vi "000_LaunchPanel.vi"(11 "Queue Ref In":T1={"UI"=refnum, "Message"=refnum, "Data"=refnum, "Caller"=refnum, "Name"="000 Common", "Data Path"=path "", "Class Path"=path "", "SubPanel"=refnum, "Project Name"="", "MNT"="", "Title"="", "Data Source"=refnum, "Queue List"={}, "VI"=refnum, "UE"=refnum}) -> ()   [LabVIEW 2020]
doc: "000001"
uses:
  Alin/QMH/000 Module Data Type.ctl
  Alin/QMH/Queue Message.ctl
panel:
  out "Tips":string
  out "Title":u8(slide) scale=0.0..100.0
  # "欢迎使用AlinFramework"
  # "加油小林哥Bilibili"
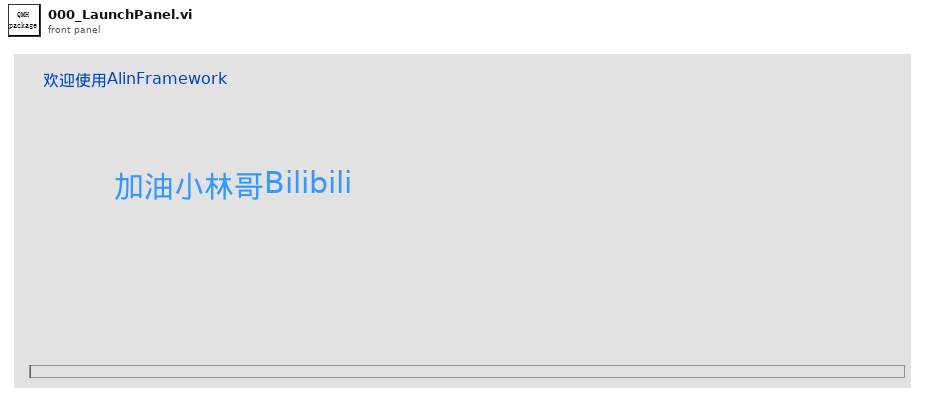
[diagram p1: front panel]
types:
  T1 = typedef "000 Module Data Type.ctl" = cluster{"UI":refnum<queue>, "Message":refnum<queue>, "Data":refnum<queue>, "Caller":refnum<queue>, "Name":string, "Data Path":path, "Class Path":path, "SubPanel":refnum<vi>, "Project Name":string, "MNT":string, "Title":string, "Data Source":refnum<queue>, "Queue List":map{string, refnum<queue>}, "VI":refnum<vi>, "UE":refnum<user-event>}
  T2 = cluster{"Queue":T1, "Delay":cluster{"Count Time(ms)":u32, "Delay Time(ms)":u32, "Next":string, "Restart":bool}}
  T3 = enum32{"Invalid", "Standard", "Closed", "Hidden", "Minimized", "Maximized"}
  T4 = typedef "eventvkey.ctl" = enum16{"ASCII", "Enter", "Return", "Shift", "Ctrl", "Alt", "Cmd", "Opt", "Caps", "NumLock", "Clear", "Break", "Up", "Down", "Left", "Right", "Insert", "Delete", "Home", "End", "PageUp", "PageDown", "Escape", "Help", "Pause", "ScrollLock", "F1", "F2", "F3", "F4", "F5", "F6", "F7", "F8", "F9", "F10", "F11", "F12", "F13", "F14", "F15", "F16", "F17", "F18", "F19", "F20", "F21", "F22", "F23", "F24", "Play", "VolumeUp", "VolumeDown", "Mute", "Two Byte Char"}
  T5 = cluster{"Shift":bool, "Ctrl":bool, "Alt":bool, "Cmd":bool, "Opt":bool}
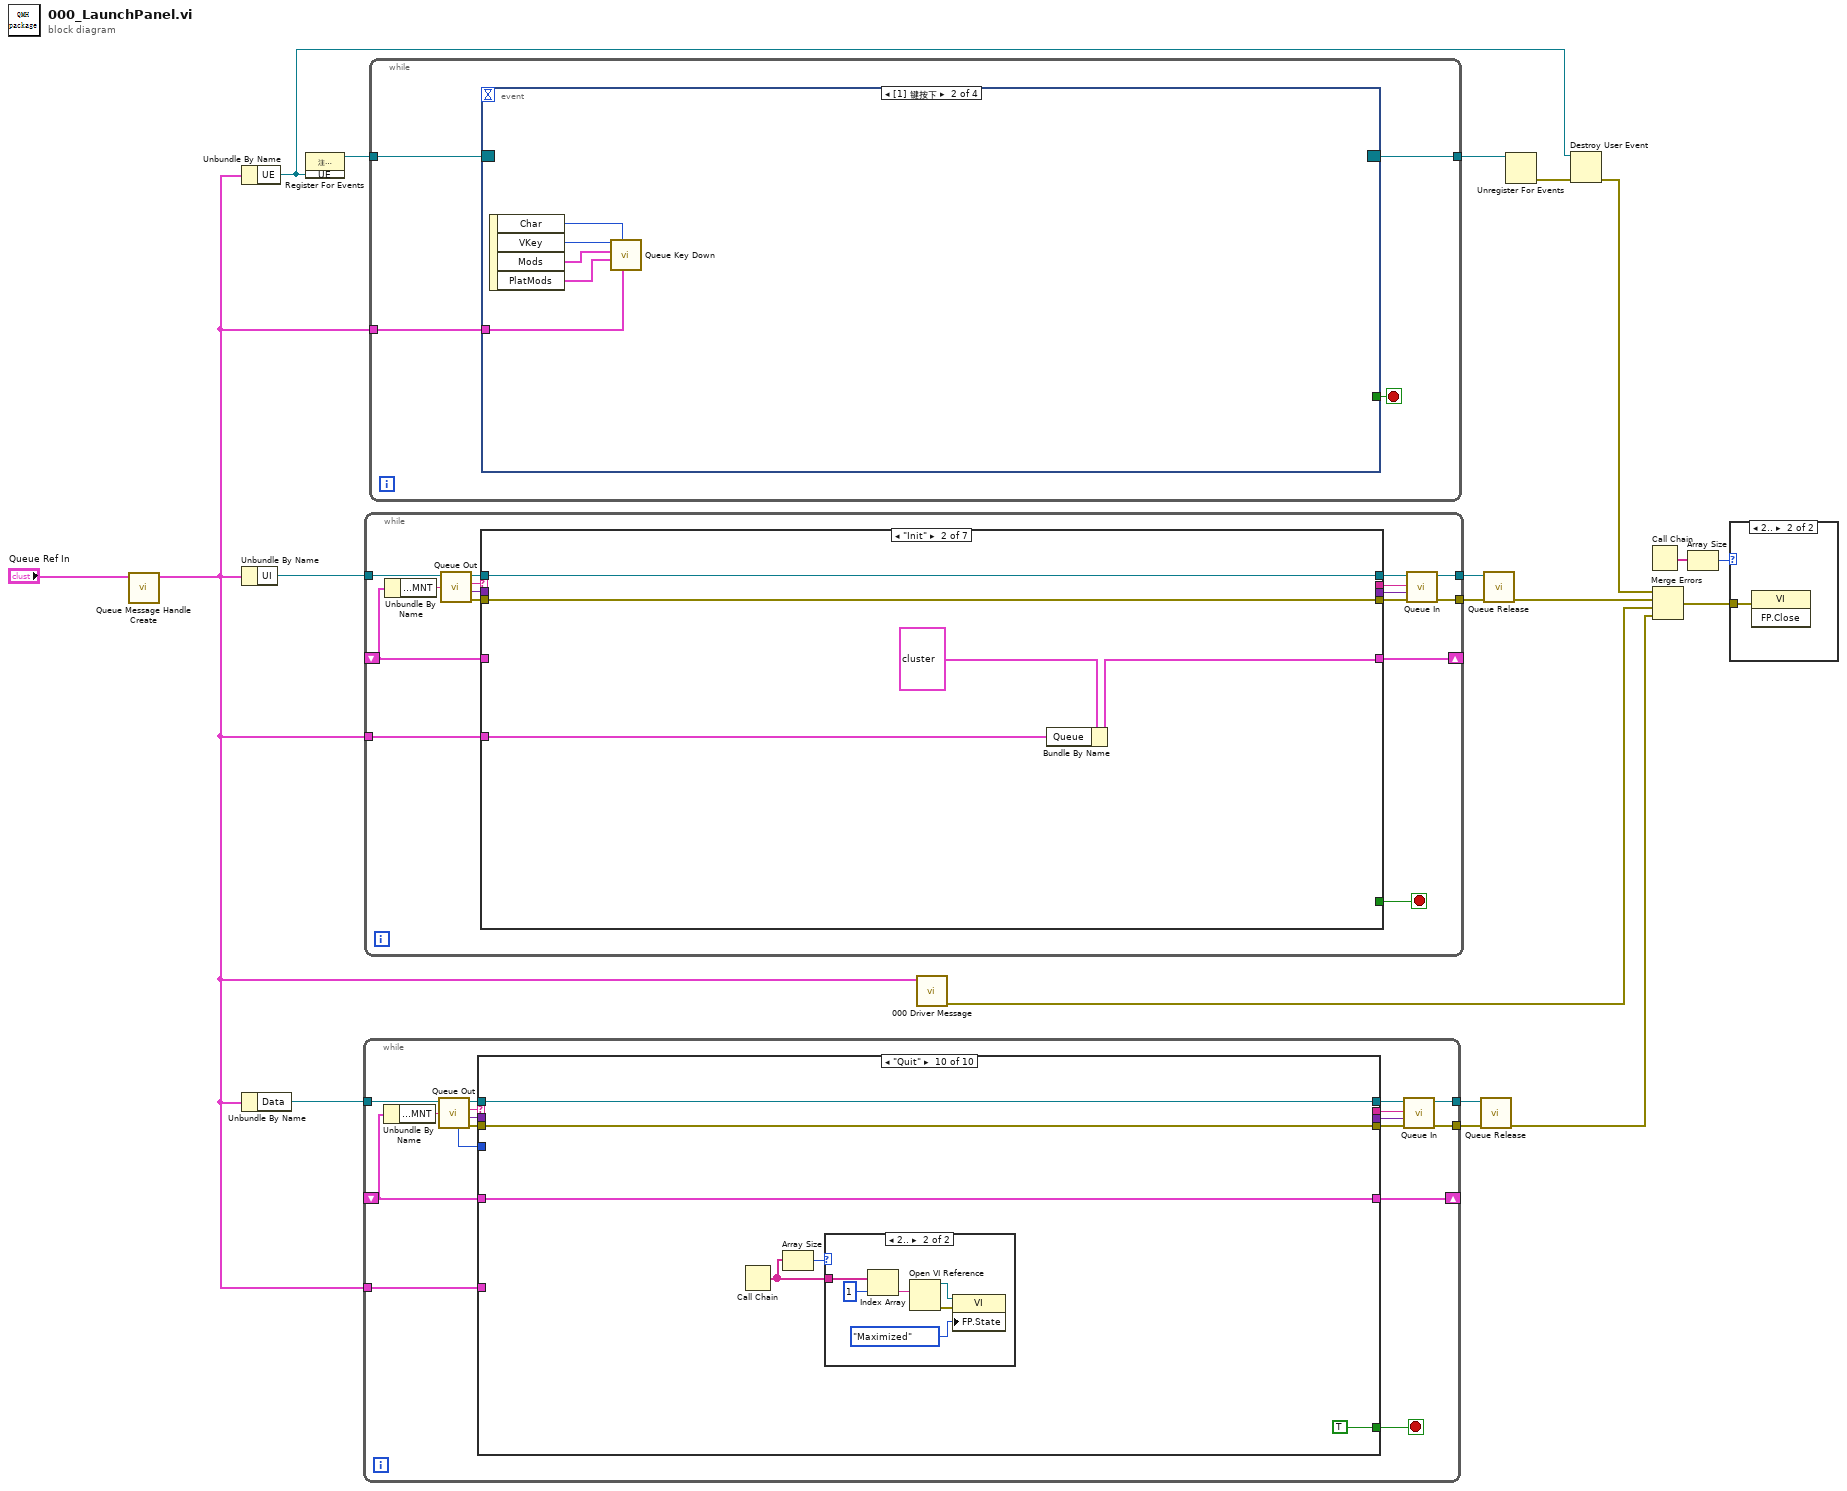
[diagram p0: block diagram]
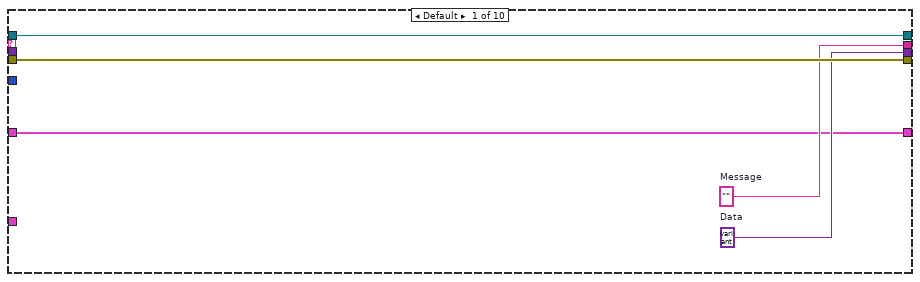
[diagram p2: hidden frame]
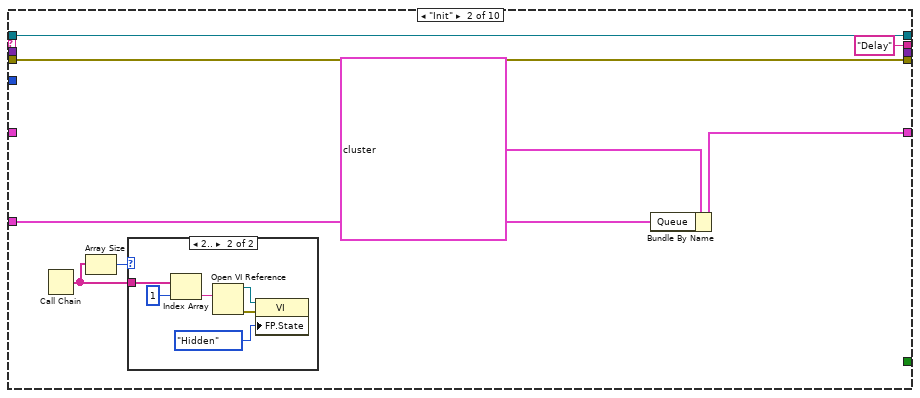
[diagram p3: hidden frame]
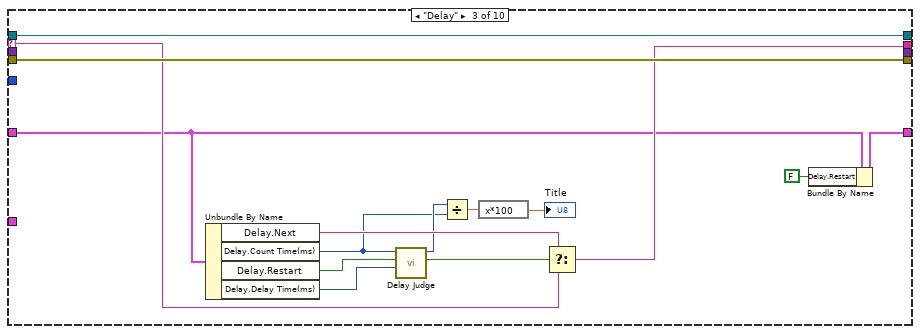
[diagram p5: hidden frame]
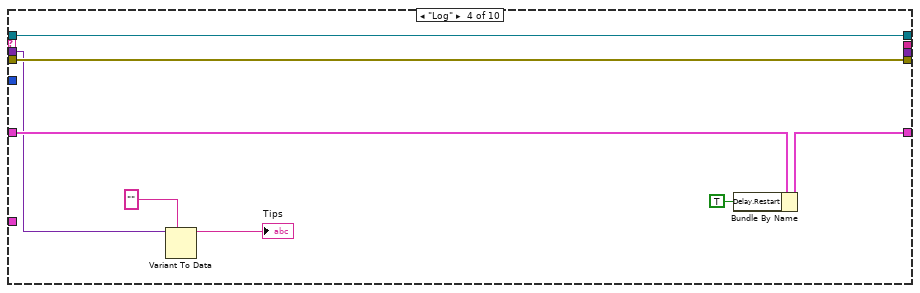
[diagram p6: hidden frame]
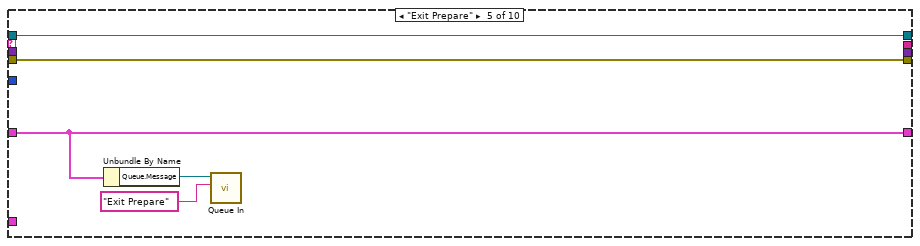
[diagram p7: hidden frame]
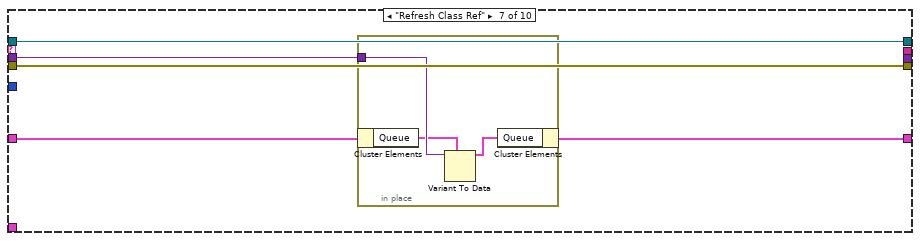
[diagram p9: hidden frame]
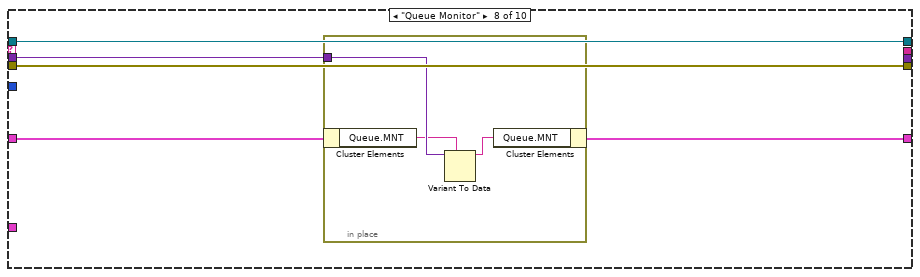
[diagram p10: hidden frame]
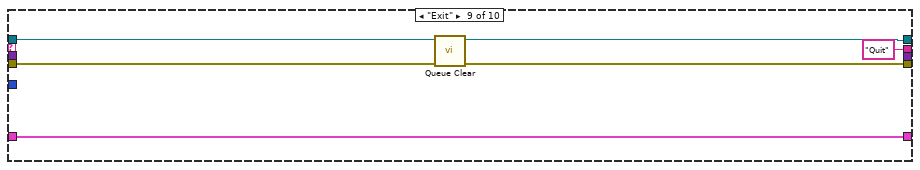
[diagram p11: hidden frame]
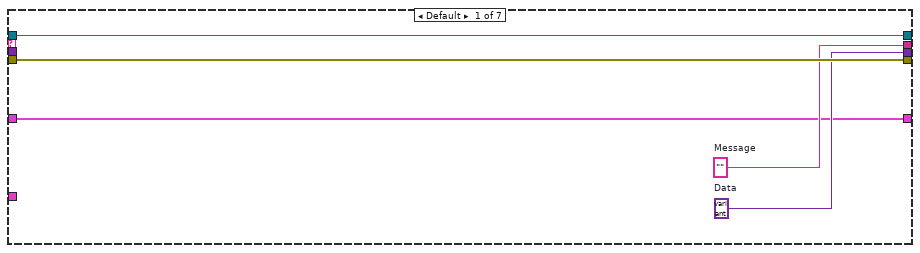
[diagram p14: hidden frame]
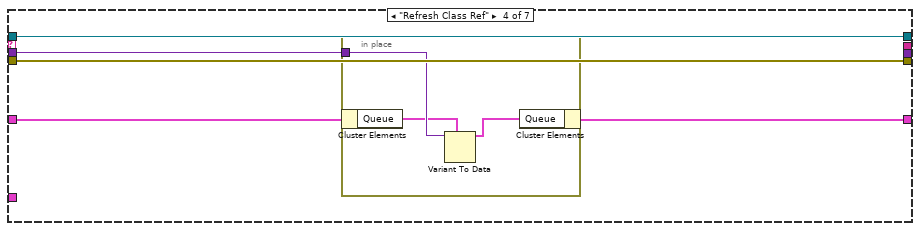
[diagram p16: hidden frame]
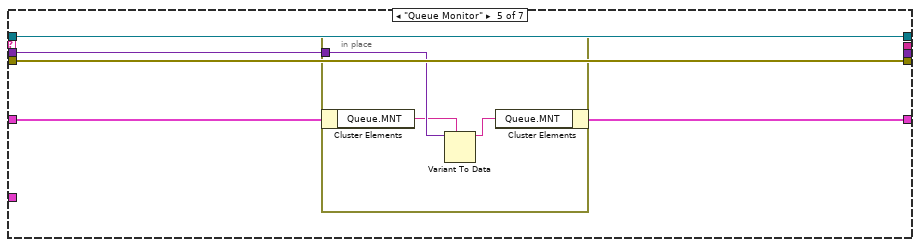
[diagram p17: hidden frame]
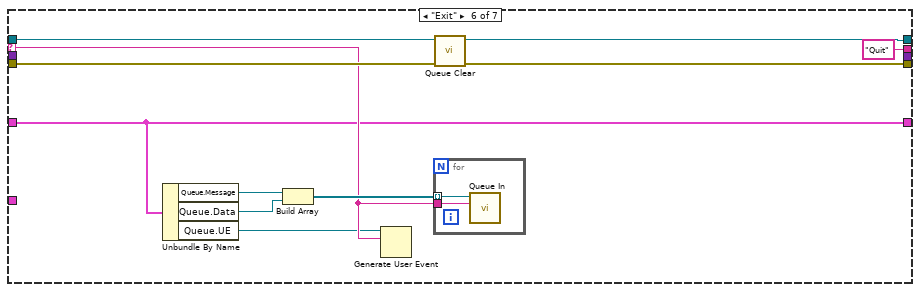
[diagram p18: hidden frame]
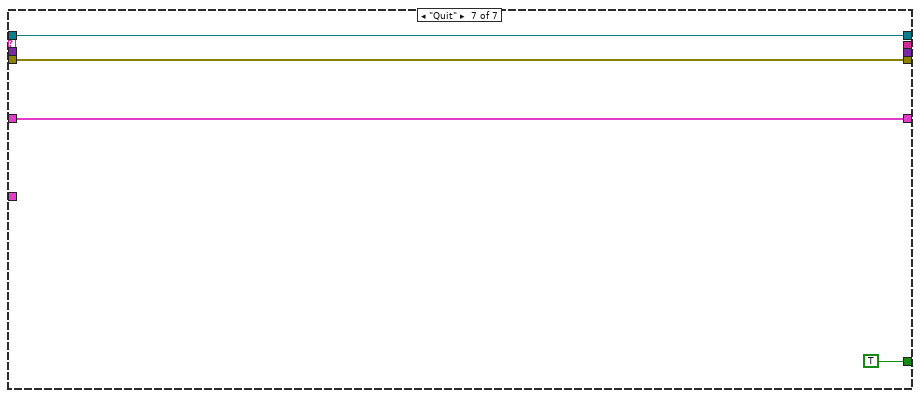
[diagram p19: hidden frame]
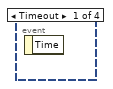
[diagram p20: hidden frame]
diagram:
  n1 = call "Queue Message Handle Create.vi"("Queue Ref In"="Queue Ref In") -> ("Queue Ref Out"=w1:T1)  [unwired: 9 in, 1 out]
  n2 = Unbundle By Name(w1) -> ("UE"=w3:refnum<user-event>)
  n3 = Unbundle By Name(w1) -> ("UI"=w14:refnum<queue>)
  n4 = Unbundle By Name(w1) -> ("Data"=w6:refnum<queue>)
  n5 = register-events(w3) -> (reference out=w19:refnum<event-registration>)  [unwired: 2 in, 1 out]
  n6 = while {
    tunnel: w6 -> [w32]
    tunnel: [w29] -> w8
    tunnel: [w28] -> w7
    shift-right: [w24] -> _
    shift-left: _ -> [w21]
    tunnel: w1 -> [w20]
    stop <- w36 stop-if-true
    n7 = Unbundle By Name(w21) -> ("Queue.MNT"=w22:string)
    n8 = call "Queue Out.vi"("Monitor"=w22, "Queue In"=w32) -> ("error out"=w35:errorcluster, "Data"=w33:variant, "Message"=w34:string, "Queue Out"=w31:refnum<queue>, "Queue NUmber"=w23:i32)  [unwired: 5 in]
    n9 = case shown="\"Quit\"" w34 {
      selector: w34 -> [_ _ w65 _ _ _ _ _ _ _]
      tunnel: w31 -> [w41 w49 w70 w78 w83 w86 w91 w99 w107 w113]
      tunnel: w35 -> [w40 w48 w69 w77 w82 w85 w90 w98 w105 w114]
      tunnel: [w41 w49 w70 w78 w83 w86 w91 w99 w106 w113] -> w30
      tunnel: [w40 w48 w69 w77 w82 w85 w90 w98 w104 w114] -> w27
      tunnel: [w39 "Delay" ("Next") w66 _ _ _ _ _ "Quit" _] -> w26
      tunnel: [_ _ _ _ _ _ _ _ _ TRUE] -> w36
      tunnel: [w38 _ _ _ _ _ _ _ _ _] -> w25
      tunnel: w33 -> [_ _ _ w73 _ _ w87 w95 _ _]
      tunnel: [w37 w45 w61 w75 w81 w84 w88 w96 w103 w111] -> w24
      tunnel: w21 -> [w37 _ w64 w76 w81 w84 w89 w97 w103 w111]
      tunnel: w23 -> [_ _ _ _ _ _ _ _ _ _]
      tunnel: w20 -> [_ w44 _ _ _ _ _ _ _ _]
      frame Default {
        w38 = variant  # Data
        w39 = ""  # Message
      }
      frame "Init" {
        n10 = Call Chain() -> (call chain=w42:string[])
        n11 = Array Size(array=w42) -> (size(s)=w43:i32)
        n12 = case shown="2.." w43 {
          tunnel: w42 -> [_ w50]
          frame 0, Default {
          }
          frame 2.. {
            n13 = Index Array(array=w50, index=1 ("索引")) -> (element=w53:string)
            n14 = Open VI Reference(vi path=w53) -> (vi reference=w54:refnum<vi>, error out=w55:errorcluster)  [unwired: 5 in]
            n15 = property class="VI"(reference=w54, error in=w55, "FP.State"=T3."Hidden" ("前面板窗口:状态")) -> ()  [unwired: 2 out]
          }
        }
        n16 = Bundle By Name(cluster=T2 {"Queue"={"UI"=refnum, "Message"=refnum, "Data"=refnum, "Caller"=refnum, "Name"="000 Common", "Data Path"=path "", "Class Path"=path "", "SubPanel"=refnum, "Project Name"="", "MNT"="", "Title"="", "Data Source"=refnum, "Queue List"={}, "VI"=refnum, "UE"=refnum}, "Delay"={"Count Time(ms)"=2000, "Delay Time(ms)"=10, "Next"="Exit Prepare,Delay", "Restart"=FALSE}}, "Queue"=w44) -> (w45:T2)
      }
      frame "Delay" {
        n17 = Unbundle By Name(w64) -> ("Delay.Next"=w68:string, "Delay.Count Time(ms)"=w57:u32, "Delay.Restart"=w63:bool, "Delay.Delay Time(ms)"=w62:u32)
        n18 = call "Delay Judge.vi"("Delay Time(ms)"=w62, "Restart"=w63, "Count Time(ms)"=w57) -> ("Time Out?"=w67:bool, "Elapsed time(ms)"=w58:u32)  [unwired: 4 in, 3 out]
        n19 = Divide(x=w58, y=w57) -> (x/y=w59:dbl)
        n20 = expression code="x*100"(w59) -> (→"Title":dbl)
        n21 = Select(t=w68, s=w67, f=w65) -> (s? t:f=w66:string)
        n22 = Bundle By Name(cluster=w64, "Delay.Restart"=FALSE) -> (w61:T2)
      }
      frame "Log" {
        n23 = Variant To Data(type="", Variant=w73) -> (data=→"Tips":string)  [unwired: 1 in, 1 out]
        n24 = Bundle By Name(cluster=w76, "Delay.Restart"=TRUE) -> (w75:T2)
      }
      frame "Exit Prepare" {
        n25 = Unbundle By Name(w81) -> ("Queue.Message"=w80:refnum<queue>)
        n26 = call "Queue In.vi"("Message"="Exit Prepare", "Queue In"=w80) -> ()  [unwired: 8 in, 2 out]
      }
      frame "====System====" {
      }
      frame "Refresh Class Ref" {
        n27 = in-place {
          in-place-border: w87 -> [w94]
          n28 = in-place-cluster #1(w89) -> ("Queue"=w93:T1)
          n29 = Variant To Data(type=w93, Variant=w94) -> (data=w92:T1)  [unwired: 1 in, 1 out]
          n30 = in-place-cluster #1("Queue"=w92) -> (w88:T2)
        }
      }
      frame "Queue Monitor" {
        n31 = in-place {
          in-place-border: w95 -> [w102]
          n32 = in-place-cluster #2(w97) -> ("Queue.MNT"=w101:string)
          n33 = Variant To Data(type=w101, Variant=w102) -> (data=w100:string)  [unwired: 1 in, 1 out]
          n34 = in-place-cluster #2("Queue.MNT"=w100) -> (w96:T2)
        }
      }
      frame "Exit" {
        n35 = call "Queue Clear.vi"("error in (no error)"=w105, "Queue In"=w107) -> ("error out"=w104:errorcluster, "Queue Out"=w106:refnum<queue>)  [unwired: 8 in]
      }
      frame "Quit" {
        n36 = Call Chain() -> (call chain=w109:string[])
        n37 = Array Size(array=w109) -> (size(s)=w110:i32)
        n38 = case shown="2.." w110 {
          tunnel: w109 -> [_ w115]
          frame 0, Default {
          }
          frame 2.. {
            n39 = Index Array(array=w115, index=1 ("索引")) -> (element=w118:string)
            n40 = Open VI Reference(vi path=w118) -> (vi reference=w119:refnum<vi>, error out=w120:errorcluster)  [unwired: 5 in]
            n41 = property class="VI"(reference=w119, error in=w120, "FP.State"=T3."Maximized" ("前面板窗口:状态")) -> ()  [unwired: 2 out]
          }
        }
      }
    }
    n42 = call "Queue In.vi"("error in (no error)"=w27, "Data"=w25, "Message"=w26, "Queue In"=w30) -> ("error out"=w28:errorcluster, "Queue Out"=w29:refnum<queue>)  [unwired: 6 in]
  }
  n43 = while {
    tunnel: w14 -> [w132]
    tunnel: [w129] -> w16
    tunnel: [w128] -> w15
    shift-right: [w124] -> _
    shift-left: _ -> [w123]
    tunnel: w1 -> [w121]
    stop <- w136 stop-if-true
    n44 = Unbundle By Name(w123) -> ("Queue.MNT"=w122:string)
    n45 = call "Queue Out.vi"("Monitor"=w122, "Queue In"=w132) -> ("error out"=w135:errorcluster, "Data"=w133:variant, "Message"=w134:string, "Queue Out"=w131:refnum<queue>)  [unwired: 5 in, 1 out]
    n46 = case shown="\"Init\"" w134 {
      selector: w134 -> [_ _ _ _ _ w168 _]
      tunnel: w131 -> [w141 w146 w149 w154 w162 w175 w181]
      tunnel: w135 -> [w140 w145 w148 w153 w161 w173 w182]
      tunnel: [w141 w146 w149 w154 w162 w174 w181] -> w130
      tunnel: [w140 w145 w148 w153 w161 w172 w182] -> w127
      tunnel: [w139 _ _ _ _ "Quit" _] -> w126
      tunnel: [_ _ _ _ _ _ TRUE] -> w136
      tunnel: [w138 _ _ _ _ _ _] -> w125
      tunnel: w133 -> [_ _ _ w150 w158 _ _]
      tunnel: [w137 w143 w147 w151 w159 w167 w179] -> w124
      tunnel: w123 -> [w137 _ w147 w152 w160 w167 w179]
      tunnel: w121 -> [_ w142 _ _ _ _ _]
      frame Default {
        w138 = variant  # Data
        w139 = ""  # Message
      }
      frame "Init" {
        n47 = Bundle By Name(cluster=cluster{"Queue":T1} {"Queue"={"UI"=refnum, "Message"=refnum, "Data"=refnum, "Caller"=refnum, "Name"="000 Common", "Data Path"=path "", "Class Path"=path "", "SubPanel"=refnum, "Project Name"="", "MNT"="", "Title"="", "Data Source"=refnum, "Queue List"={}, "VI"=refnum, "UE"=refnum}}, "Queue"=w142) -> (w143:cluster{"Queue":T1})
      }
      frame "====System====" {
      }
      frame "Refresh Class Ref" {
        n48 = in-place {
          in-place-border: w150 -> [w157]
          n49 = in-place-cluster #3(w152) -> ("Queue"=w156:T1)
          n50 = Variant To Data(type=w156, Variant=w157) -> (data=w155:T1)  [unwired: 1 in, 1 out]
          n51 = in-place-cluster #3("Queue"=w155) -> (w151:cluster{"Queue":T1})
        }
      }
      frame "Queue Monitor" {
        n52 = in-place {
          in-place-border: w158 -> [w165]
          n53 = in-place-cluster #4(w160) -> ("Queue.MNT"=w164:string)
          n54 = Variant To Data(type=w164, Variant=w165) -> (data=w163:string)  [unwired: 1 in, 1 out]
          n55 = in-place-cluster #4("Queue.MNT"=w163) -> (w159:cluster{"Queue":T1})
        }
      }
      frame "Exit" {
        n56 = Unbundle By Name(w167) -> ("Queue.Message"=w171:refnum<queue>, "Queue.Data"=w170:refnum<queue>, "Queue.UE"=w166:refnum<user-event>)
        n57 = Build Array(w171, w170) -> (w169:refnum<queue>[])
        n58 = Generate User Event(user event=w166, event data cluster=w168) -> ()  [unwired: 2 in, 2 out]
        n59 = for {
          tunnel: w169 -> [w178] mode=indexing
          tunnel: w168 -> [w177]
          n60 = call "Queue In.vi"("Message"=w177, "Queue In"=w178) -> ()  [unwired: 8 in, 2 out]
        }
        n61 = call "Queue Clear.vi"("error in (no error)"=w173, "Queue In"=w175) -> ("error out"=w172:errorcluster, "Queue Out"=w174:refnum<queue>)  [unwired: 8 in]
      }
      frame "Quit" {
      }
    }
    n62 = call "Queue In.vi"("error in (no error)"=w127, "Data"=w125, "Message"=w126, "Queue In"=w130) -> ("error out"=w128:errorcluster, "Queue Out"=w129:refnum<queue>)  [unwired: 6 in]
  }
  n63 = while {
    tunnel: w19 -> [w186]
    tunnel: [w184] -> w18
    tunnel: w1 -> [w183]
    stop <- w185 stop-if-true
    n64 = event shown="[1] 键按下" {
      selector: w186 -> [_ _ _ _]
      dyn-events: [_ _ _ _] -> w184
      timeout: _ -> [_ _ _ _]
      tunnel: [_ _ w192 _] -> w185
      tunnel: w183 -> [_ w190 _ w197]
      event Timeout {
        n65 = event-data() -> ()  [unwired: 1 in, 1 out]
      }
      event Key Down {
        n66 = event-data() -> ("Char"=w191:i16, "VKey"=w189:T4, "Mods"=w188:cluster{"Num Pad":bool, "Menu Key":bool}, "PlatMods"=w187:T5)  [unwired: 1 in]
        n67 = call "Queue Key Down.vi"("Queue Ref Out"=w190, "C"=w191, "Platform Key"=w187, "Group Key"=w188, "V Key"=w189) -> ()  [unwired: 6 in, 1 out]
      }
      event User Event {
        n68 = event-data() -> ("Message"=w194:string)  [unwired: 1 in]
        n69 = Equal?(x=w194, y="Exit") -> (x = y?=w192:bool)
      }
      event Panel Close? {
        n70 = event-data() -> ()  [unwired: 1 in, 1 out]
        n71 = Call Chain() -> (call chain=w199:string[])
        n72 = Array Size(array=w199) -> (size(s)=w198:i32)
        n73 = case shown="2, 默认" w198 {
          tunnel: w197 -> [w203 w206]
          tunnel: [w202 w205] -> w196
          tunnel: ["Panel Hidden" ("Message") "Exit Prepare" ("Message")] -> w195
          frame 2, Default {
            n74 = Unbundle By Name(w203) -> ("Message"=w202:refnum<queue>)
          }
          frame 1 {
            n75 = Unbundle By Name(w206) -> ("Message"=w205:refnum<queue>)
          }
        }
        n76 = call "Queue In.vi"("Message"=w195, "Queue In"=w196) -> ()  [unwired: 8 in, 2 out]
        n77 = event-data("Discard?"=TRUE ("放弃？")) -> ()  [unwired: 1 in, 1 out]
      }
    }
  }
  n78 = call "000 Driver Message.vi"("Queue In"=w1) -> ("error out"=w4:errorcluster)  [unwired: 8 in, 2 out]
  n79 = call "Queue Release.vi"("error in (no error)"=w7, "Queue In"=w8) -> ("error out"=w5:errorcluster)  [unwired: 9 in]
  n80 = call "Queue Release.vi"("error in (no error)"=w15, "Queue In"=w16) -> ("error out"=w12:errorcluster)  [unwired: 9 in]
  n81 = Unregister For Events(event registration refnum=w18) -> (error out=w17:errorcluster)  [unwired: 1 in]
  n82 = Destroy User Event(user event=w3, error in=w17) -> (error out=w13:errorcluster)
  n83 = Call Chain() -> (call chain=w10:string[])
  n84 = Merge Errors(w13, w12, w4, w5) -> (w11:errorcluster)
  n85 = Array Size(array=w10) -> (size(s)=w9:i32)
  n86 = case shown="2.." w9 {
    tunnel: w11 -> [_ w207]
    frame 0, Default {
    }
    frame 2.. {
      n87 = invoke class="VI" method="FP.Close"(error in=w207) -> ()  [unwired: 2 in, 3 out]
    }
  }
